vi "Read Power-up Settings and Special Control Range.vi"(7 "Unit ID (A)":string="A", 8 "error in":errorcluster, 11 "VISA Session In":refnum<visa-resource-name>="Alicat") -> (0 "error out":errorcluster, 2 "Power-up settings & special control range":T1={"Serial/Local Setpoint"=enum."Save", "FP Buttons"=enum."Unlocked", "Valve Hard Zero"=enum."On zero setpoint", "Initial Screen"=enum."Main", "Gas Select"=enum."Save", "Tare Delay"=nan, "Control Range"=enum."Unknown"}, 3 "VISA Session Out":refnum<visa-resource-name>)   [LabVIEW 2024]
doc: "Queries the Alicat Scientific device for power-up options related to retention of setting changes, front panel display and buttons, valve zeroing, tareing, and controller range.\n\nIF WRITING MULTIPLE SETPOINTS PER SECOND: DISABLE SAVING SERIAL/LOCAL SETPOINTS TO PREVENT BURNING OUT THE EEPROM OF THE ALICAT DEVICE."
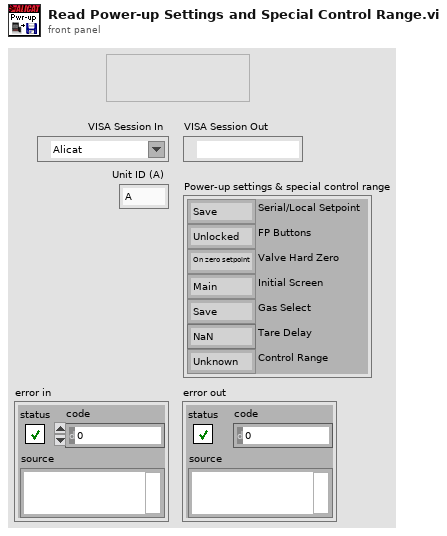
[diagram p1: front panel]
types:
  T1 = cluster{"Serial/Local Setpoint":enum8{"Don't Save", "Save"}, "FP Buttons":enum8{"Unlocked", "Locked"}, "Valve Hard Zero":enum16{"On zero setpoint", "Startup only"}, "Initial Screen":enum16{"Main", "Totalizer"}, "Gas Select":enum8{"Don't Save", "Save"}, "Tare Delay":dbl, "Control Range":enum16{"Normal", "Inverted", "Bidirectional", "Unknown"}}
  T2 = enum16{"Normal", "Inverted", "Bidirectional", "Unknown"}
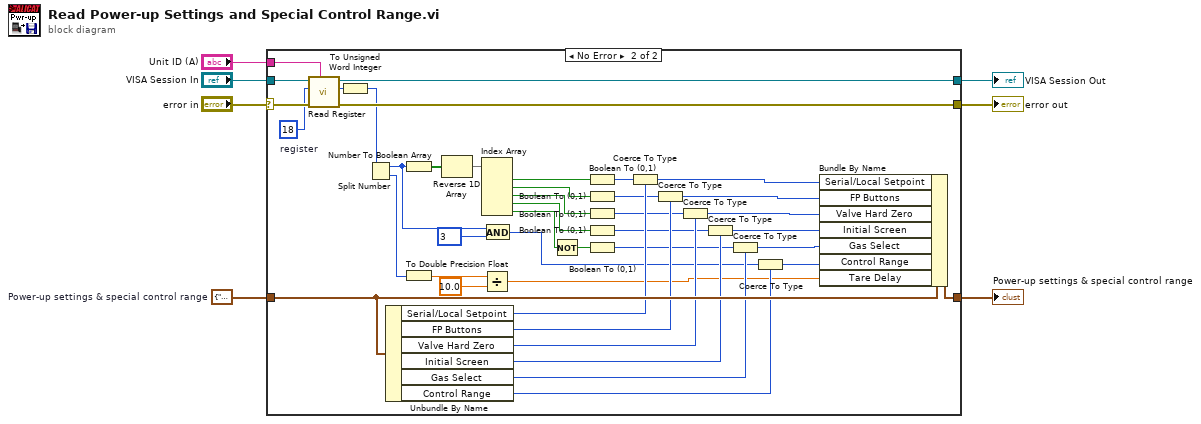
[diagram p0: block diagram]
diagram:
  w1 = T1 {"Serial/Local Setpoint"=enum."Save", "FP Buttons"=enum."Unlocked", "Valve Hard Zero"=enum."On zero setpoint", "Initial Screen"=enum."Main", "Gas Select"=enum."Save", "Tare Delay"=nan, "Control Range"=enum."Unknown"}  # Power-up settings & special control range
  n1 = case shown="No Error" "error in" {
    selector: "error in" -> [w8 w18]
    tunnel: [w10 w52] -> w2
    tunnel: w1 -> [w10 w51]
    tunnel: "VISA Session In" -> [w9 w17]
    tunnel: [w8 w16] -> w5
    tunnel: [w9 w15] -> w4
    tunnel: "Unit ID (A)" -> [_ w14]
    frame Error {
    }
    frame No Error {
      w13 = u16 18  # register
      n2 = call "Read Register.vi"("Unit ID (A)"=w14, "error in"=w18, "Register address"=w13, "VISA Session In"=w17) -> ("error out"=w16:errorcluster, "Register Value (I32)"=w11:i32, "VISA Session Out"=w15:refnum<visa-resource-name>)  [unwired: 5 in]
      n3 = To Unsigned Word Integer(number=w11) -> (unsigned 16bit integer=w12:u16)
      n4 = Split Number(x=w12) -> (hi(x)=w22:u8, lo(x)=w50:u8)
      n5 = Unbundle By Name(w51) -> ("Serial/Local Setpoint"=w43:enum8{"Don't Save", "Save"}, "FP Buttons"=w39:enum8{"Unlocked", "Locked"}, "Valve Hard Zero"=w36:enum16{"On zero setpoint", "Startup only"}, "Initial Screen"=w49:enum16{"Main", "Totalizer"}, "Gas Select"=w47:enum8{"Don't Save", "Save"}, "Control Range"=w45:T2)
      n6 = Number To Boolean Array(number=w22) -> (Boolean array=w34:bool[])
      n7 = To Double Precision Float(number=w50) -> (double precision float=w32:dbl)
      n8 = Reverse 1D Array(array=w34) -> (reversed array=w33:bool[])
      n9 = Index Array(array=w33) -> (element #1=w30:bool, element #2=w29:bool, element #3=w28:bool, element #4=w27:bool, element #5=w23:bool)  [unwired: 5 in]
      n10 = Divide(x=w32, y=10.0) -> (x/y=w24:dbl)
      n11 = And(x=w22, y=u8 3) -> (x .and. y?=w20:u8)
      n12 = Not(x=w23) -> (.not. x?=w19:bool)
      n13 = Boolean To (0,1)(Boolean=w30) -> (0, 1=w42:i16)
      n14 = Boolean To (0,1)(Boolean=w29) -> (0, 1=w40:i16)
      n15 = Boolean To (0,1)(Boolean=w28) -> (0, 1=w37:i16)
      n16 = Boolean To (0,1)(Boolean=w27) -> (0, 1=w26:i16)
      n17 = Boolean To (0,1)(Boolean=w19) -> (0, 1=w25:i16)
      n18 = Coerce To Type(0:w42, 1:w43) -> (2:w41:enum8{"Don't Save", "Save"})
      n19 = Coerce To Type(0:w40, 1:w39) -> (2:w38:enum8{"Unlocked", "Locked"})
      n20 = Coerce To Type(0:w37, 1:w36) -> (2:w35:enum16{"On zero setpoint", "Startup only"})
      n21 = Coerce To Type(0:w26, 1:w49) -> (2:w48:enum16{"Main", "Totalizer"})
      n22 = Coerce To Type(0:w25, 1:w47) -> (2:w46:enum8{"Don't Save", "Save"})
      n23 = Coerce To Type(0:w20, 1:w45) -> (2:w44:T2)
      n24 = Bundle By Name(cluster=w51, "Serial/Local Setpoint"=w41, "FP Buttons"=w38, "Valve Hard Zero"=w35, "Initial Screen"=w48, "Gas Select"=w46, "Control Range"=w44, "Tare Delay"=w24) -> (w52:T1)
    }
  }
  "error out" <- w5
  "VISA Session Out" <- w4
  "Power-up settings & special control range" <- w2
